vi "reformat message.vi"(8 "error in (no error)":errorcluster, 11 "TCS in":refnum<class "TCS.lvclass">) -> (0 "error out":errorcluster, 3 "TCS out":refnum<class "TCS.lvclass">)   [LabVIEW 2018, in "TCS.lvclass"]
uses:
  TCS.lvclass
  <vilib>/Utility/error.llb/whitespace.ctl
  TCS.lvclass/TCS.ctl
  RxTx/RxTx.lvclass
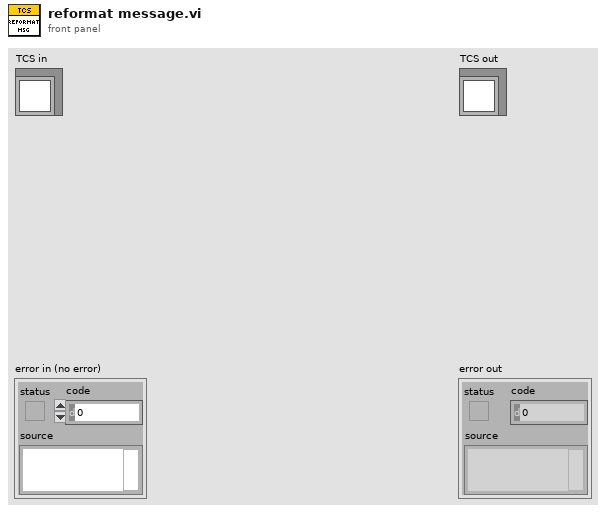
[diagram p1: front panel]
types:
  T1 = typedef "whitespace.ctl" = u16
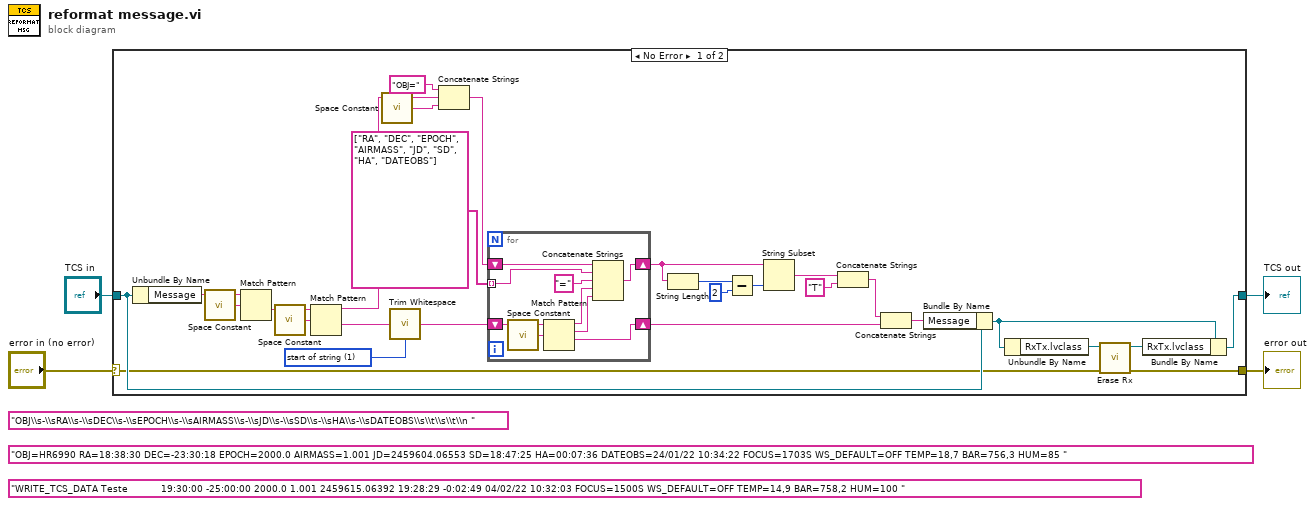
[diagram p0: block diagram]
diagram:
  (unwired) "WRITE_TCS_DATA Teste           19:30:00 -25:00:00 2000.0 1.001 2459615.06392 19:28:29 -0:02:49 04/02/22 10:32:03 FOCUS=1500S WS_DEFAULT=OFF TEMP=14,9 BAR=758,2 HUM=100 "
  (unwired) "OBJ=HR6990 RA=18:38:30 DEC=-23:30:18 EPOCH=2000.0 AIRMASS=1.001 JD=2459604.06553 SD=18:47:25 HA=00:07:36 DATEOBS=24/01/22 10:34:22 FOCUS=1703S WS_DEFAULT=OFF TEMP=18,7 BAR=756,3 HUM=85 "
  (unwired) "OBJ\\s-\\sRA\\s-\\sDEC\\s-\\sEPOCH\\s-\\sAIRMASS\\s-\\sJD\\s-\\sSD\\s-\\sHA\\s-\\sDATEOBS\\s\\t\\s\\t\\n "
  n1 = case shown="No Error" "error in (no error)" {
    selector: "error in (no error)" -> [w6 w43]
    tunnel: [w5 w43] -> w3
    tunnel: [w10 w42] -> w1
    tunnel: "TCS in" -> [w32 w42]
    frame No Error {
      w15 = T1 1 items=["both", "start of string", "end of string"] ("location (both)")
      n2 = Unbundle By Name(w32) -> ("Message"=w12:string)
      n3 = call <vilib>:"Space Constant.vi"() -> ("String"=w27:string)
      n4 = Match Pattern(string=w12, regular expression=w27) -> (after substring=w26:string)  [unwired: 1 in, 3 out]
      n5 = call <vilib>:"Space Constant.vi"() -> ("String"=w17:string)
      n6 = Match Pattern(string=w26, regular expression=w17) -> (before substring=w16:string, after substring=w14:string)  [unwired: 1 in, 2 out]
      n7 = call <vilib>:"Space Constant.vi"() -> ("String"=w30:string)
      n8 = call <vilib>:"Trim Whitespace.vi"("string"=w14, "location (both)"=w15) -> ("trimmed string"=w13:string)
      n9 = Concatenate Strings("OBJ=", w16, w30) -> (w28:string)
      n10 = for {
        tunnel: string[] ["RA", "DEC", "EPOCH", "AIRMASS", "JD", "SD", "HA", "DATEOBS"] -> [w37] mode=indexing
        shift-right: [w36] -> w18
        shift-left: w28 -> [w33]
        shift-right: [w35] -> w19
        shift-left: w13 -> [w41]
        n11 = call <vilib>:"Space Constant.vi"() -> ("String"=w40:string)
        n12 = Match Pattern(string=w41, regular expression=w40) -> (before substring=w39:string, match substring=w34:string, after substring=w35:string)  [unwired: 1 in, 1 out]
        n13 = Concatenate Strings(w33, w37, "=", w39, w34) -> (w36:string)
      }
      n14 = String Length(string=w18) -> (length=w25:i32)
      n15 = Subtract(x=w25, y=2) -> (x-y=w23:i32)
      n16 = String Subset(string=w18, length (rest)=w23) -> (substring=w22:string)  [unwired: 1 in]
      n17 = Concatenate Strings(w22, "T") -> (w20:string)
      n18 = Concatenate Strings(w20, w19) -> (w11:string)
      n19 = Bundle By Name(cluster=w32, "Message"=w11) -> (w9:refnum<class "TCS.lvclass">)
      n20 = Unbundle By Name(w9) -> ("RxTx.lvclass"=w8:refnum<class "RxTx.lvclass">)
      n21 = call "Erase Rx.vi"("error in (no error)"=w6, "RxTx in"=w8) -> ("error out"=w5:errorcluster, "RxTx out"=w7:refnum<class "RxTx.lvclass">)  [unwired: 8 in]
      n22 = Bundle By Name(cluster=w9, "RxTx.lvclass"=w7) -> (w10:refnum<class "TCS.lvclass">)
    }
    frame Error {
    }
  }
  "error out" <- w3
  "TCS out" <- w1
